vi "Arrays_Dbl Set Size.vi"(3 "Array":dbl[](array[numeric]), 4 "Size":i32) -> (5 "Array Out":dbl[](array[numeric]))   [LabVIEW 2015]
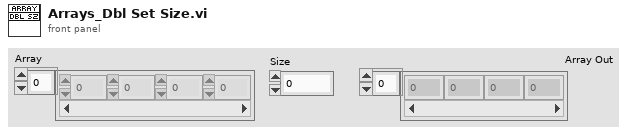
[diagram p1: front panel]
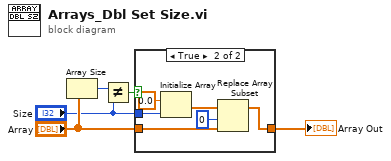
[diagram p0: block diagram]
diagram:
  n1 = Array Size(array="Array") -> (size(s)=w3:i32)
  n2 = Not Equal?(x=w3, y="Size") -> (x != y?=w1:bool)
  n3 = case shown="True" w1 {
    tunnel: [w6 w12] -> w5
    tunnel: "Size" -> [_ w8]
    tunnel: "Array" -> [w6 w7]
    frame False {
    }
    frame True {
      n4 = Initialize Array(0.0, w8) -> (w10:dbl[])
      n5 = Replace Array Subset(array=w10, new element=w7, index=0) -> (w12:dbl[])
    }
  }
  "Array Out" <- w5
